vi "DialogCreateClass_HandleTemplatesDialog.vi"(8 "error in (no error)":errorcluster, 11 "AllTemplatesForThisProvider/InheritanceType(Base/Sub)":T1[](array[typedef])) -> (0 "error out":errorcluster)   [LabVIEW 2020, in "ClassWriterNative.lvclass"]
uses:
  <resource>/Framework/Providers/Open_GDS/ClassProviders/Provider_LvNativeClass/ClassWriterNative_class/ClassWriterNative.lvclass
  <resource>/Framework/Providers/Open_GDS/ClassProviders/Provider_BaseClassInterface/ClassTemplateType.ctl
  <vilib>/Utility/config.llb/Write Key (String).vi
  <vilib>/Utility/config.llb/NI_LVConfig.lvlib
  <resource>/Framework/Providers/Open_GDS/ClassProviders/Provider_BaseClassInterface/ClassWriter_class/ClassWriter.lvclass
panel:
  in  "Cancel":bool
  in  "Save":bool
  in  "Down":bool
  in  "Up":bool
  in  "ClassTemplates":i32(listbox) caption="Class Templates"
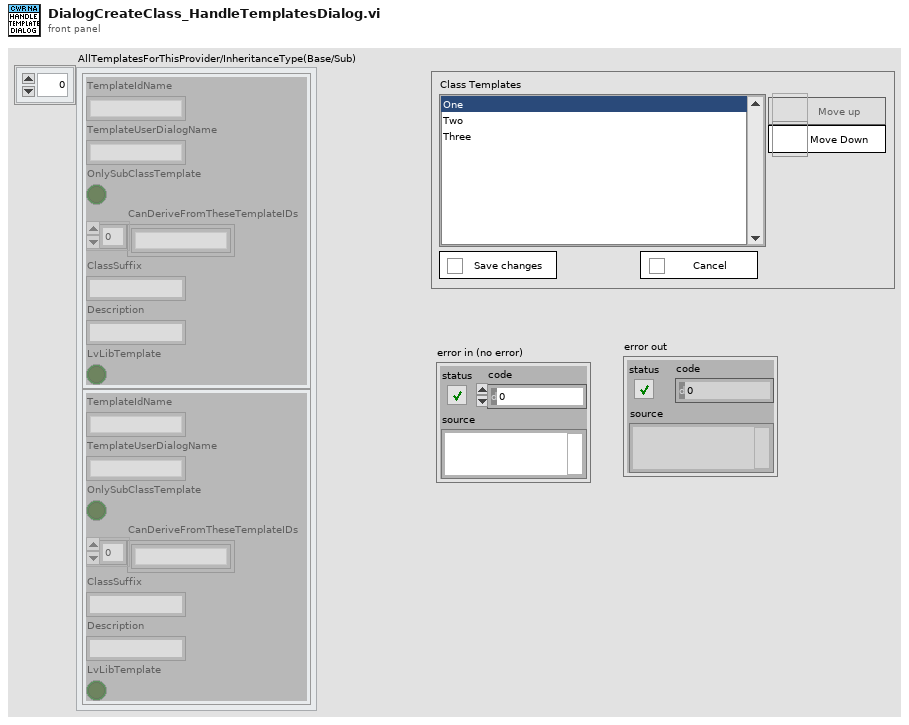
[diagram p1: front panel]
types:
  T1 = typedef "ClassWriter.lvclass/ClassTemplateType.ctl" = cluster{"TemplateIdName":string, "TemplateUserDialogName":string, "OnlySubClassTemplate":bool, "CanDeriveFromTheseTemplateIDs":string[], "ClassSuffix":string, "Description":string, "LvLibTemplate":bool}
  T2 = cluster{"FilterSettings":cluster{"Numeric":i32, "Boolean":bool}[], "Section":string}
  T3 = enum8{"Enabled", "Disabled", "Disabled and Grayed Out"}
  T4 = typedef "LVPoint32TypeDef.ctl" = cluster{"Horizontal":i32, "Vertical":i32}
  T5 = typedef "NI_LVConfig.lvlib/Config Data RefNum.ctl" = refnum<k1>
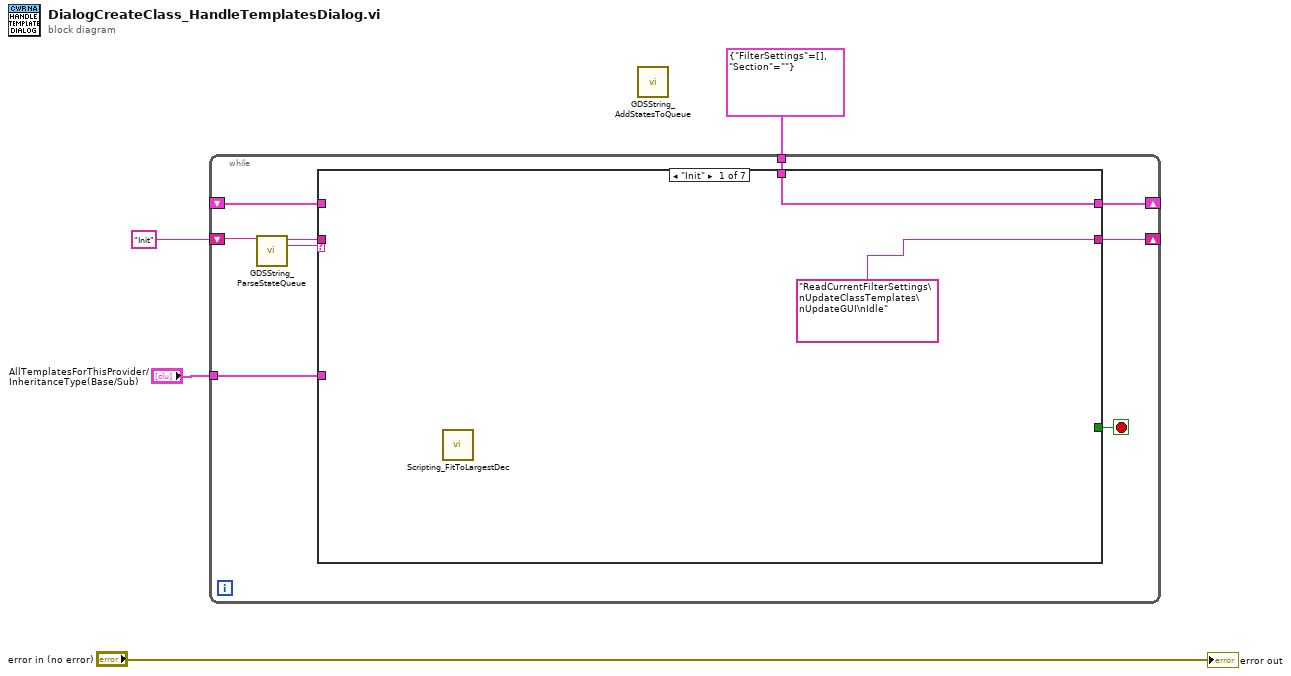
[diagram p0: block diagram]
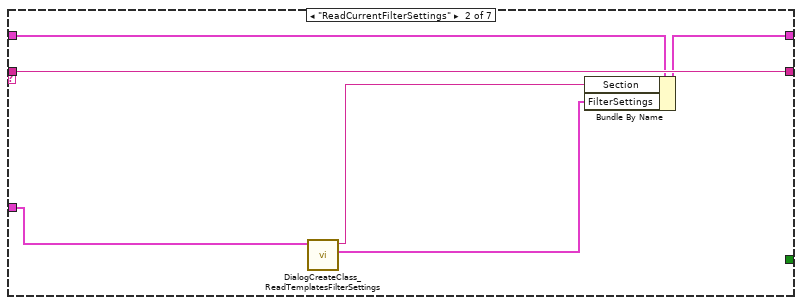
[diagram p2: hidden frame]
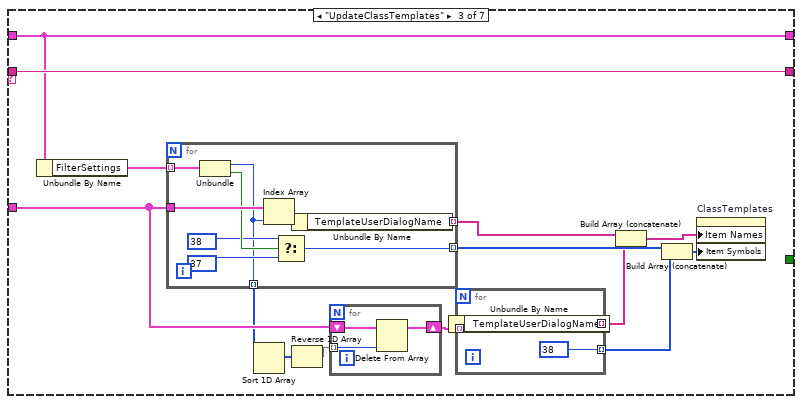
[diagram p3: hidden frame]
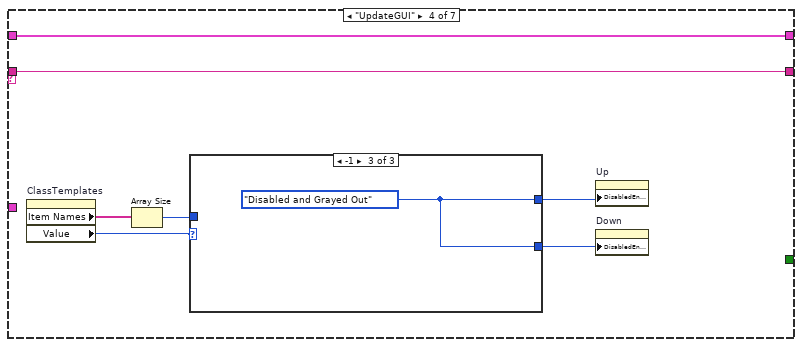
[diagram p4: hidden frame]
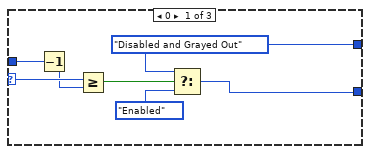
[diagram p5: hidden frame]
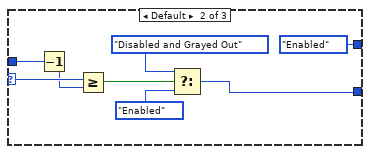
[diagram p6: hidden frame]
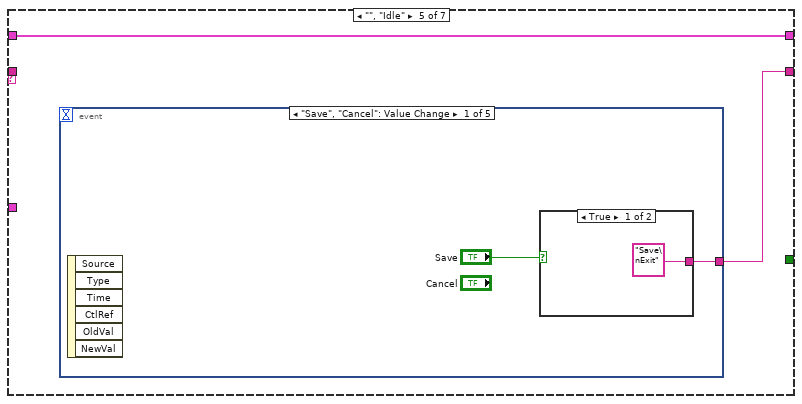
[diagram p7: hidden frame]
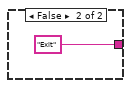
[diagram p8: hidden frame]
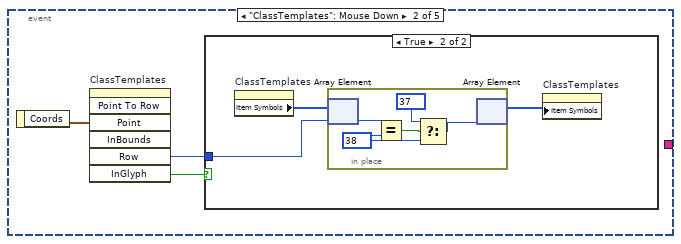
[diagram p9: hidden frame]
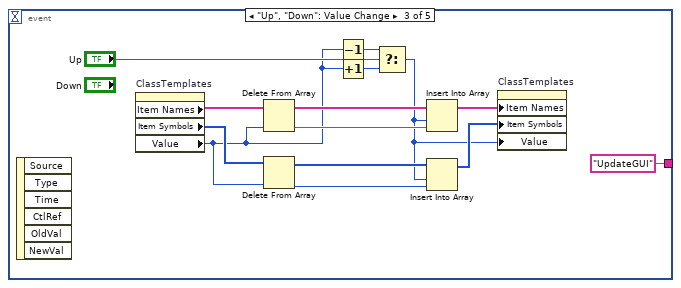
[diagram p11: hidden frame]
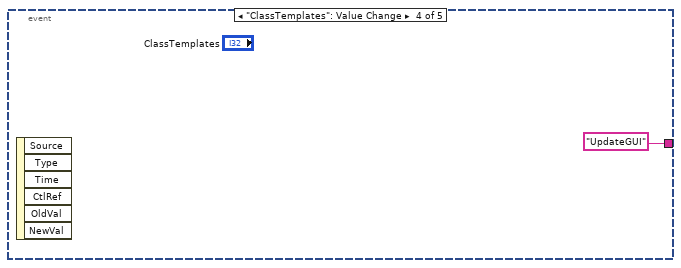
[diagram p12: hidden frame]
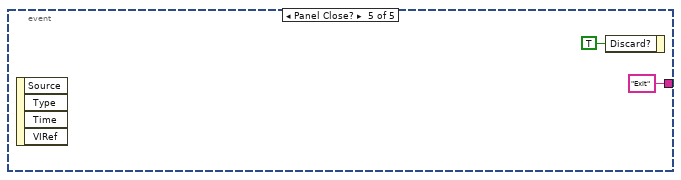
[diagram p13: hidden frame]
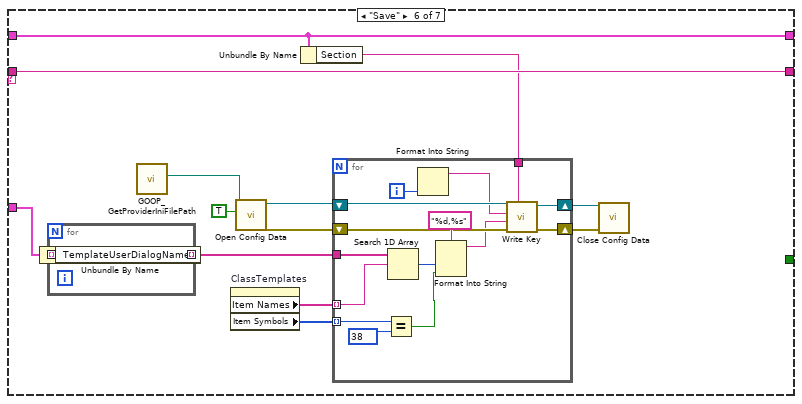
[diagram p14: hidden frame]
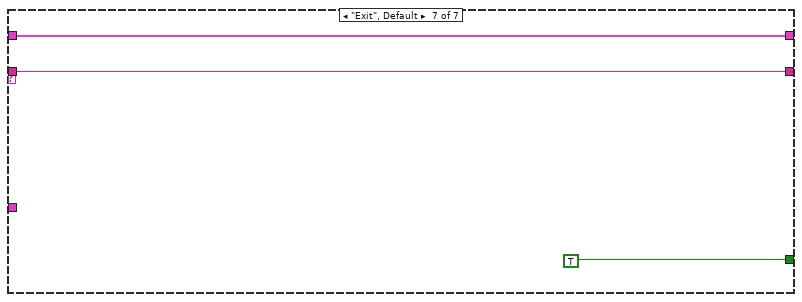
[diagram p15: hidden frame]
diagram:
  n1 = while {
    shift-right: [w11] -> _
    shift-left: "Init" -> [w12]
    tunnel: "AllTemplatesForThisProvider/InheritanceType(Base/Sub)" -> [w8]
    tunnel: T2 {"FilterSettings"=[], "Section"=""} -> [w7]
    shift-right: [w6] -> _
    shift-left: _ -> [w5]
    stop <- w13 stop-if-true
    n2 = call <resource>:"GDSString_ParseStateQueue.vi"("State Queue"=w12) -> ("Remaining States"=w9:string, "Current State"=w10:string)  [unwired: 10 in, 3 out]
    n3 = case shown="\"Init\"" w10 {
      tunnel: [_ _ _ _ _ _ TRUE] -> w13
      tunnel: ["ReadCurrentFilterSettings\nUpdateClassTemplates\nUpdateGUI\nIdle" ("Remaining States") w21 w35 w57 w75 w120 w139] -> w11
      tunnel: w9 -> [_ w21 w35 w57 _ w120 w139]
      tunnel: w8 -> [_ w20 w30 _ _ w117 _]
      tunnel: [w14 w17 w34 w56 w74 w114 w138] -> w6
      tunnel: w7 -> [w14 _ _ _ _ _ _]
      tunnel: w5 -> [_ w19 w34 w56 w74 w114 w138]
      frame "Init" {
        n4 = call <resource>:"Scripting_FitToLargestDec.vi"() -> ()  [unwired: 6 in, 2 out]
      }
      frame "ReadCurrentFilterSettings" {
        n5 = call <resource>:"DialogCreateClass_ReadTemplatesFilterSettings.vi"("AllTemplatesForThisProvider/InheritanceType(Base/Sub)"=w20) -> ("FilterSettings(OrderIndex,Active)"=w18:cluster{"Numeric":i32, "Checkbox":bool}[], "Section"=w16:string)  [unwired: 9 in]
        n6 = Bundle By Name(cluster=w19, "Section"=w16, "FilterSettings"=w18) -> (w17:T2)
      }
      frame "UpdateClassTemplates" {
        n7 = Unbundle By Name(w34) -> ("FilterSettings"=w33:cluster{"Numeric":i32, "Boolean":bool}[])
        n8 = for {
          tunnel: w33 -> [w50] mode=indexing
          tunnel: w30 -> [w49]
          tunnel: [w45] -> w32 mode=indexing
          tunnel: [w43] -> w31 mode=indexing
          tunnel: [w42] -> w29 mode=indexing
          n9 = Unbundle(w50) -> ("Numeric"=w42:i32, "Boolean"=w48:bool)
          n10 = Index Array(array=w49, index=w42) -> (element=w44:T1)
          n11 = Select(t=38, s=w48, f=37) -> (s? t:f=w45:i32)
          n12 = Unbundle By Name(w44) -> ("TemplateUserDialogName"=w43:string)
        }
        n13 = Sort 1D Array(array=w29) -> (sorted array=w28:i32[])
        n14 = Reverse 1D Array(array=w28) -> (reversed array=w27:i32[])
        n15 = for {
          shift-right: [w39] -> w26
          shift-left: w30 -> [w41]
          tunnel: w27 -> [w40] mode=indexing
          n16 = Delete From Array(array=w41, index=w40) -> (array with subset deleted=w39:T1[])  [unwired: 1 in, 1 out]
        }
        n17 = for {
          tunnel: [38] -> w22 mode=indexing
          tunnel: [w38] -> w23 mode=indexing
          tunnel: w26 -> [w36] mode=indexing
          n18 = Unbundle By Name(w36) -> ("TemplateUserDialogName"=w38:string)
        }
        n19 = Build Array (concatenate)(w31, w23) -> (w25:string[])
        n20 = Build Array (concatenate)(w32, w22) -> (w24:i32[])
        n21 = property on="ClassTemplates" class="LstBox (strict)"("Item Names"=w25, "Item Symbols"=w24) -> ()  [unwired: 2 in, 2 out]
      }
      frame "UpdateGUI" {
        n22 = property on="ClassTemplates" class="LstBox (strict)"() -> ("Item Names"=w52:string[], "Value"=w55:i32)  [unwired: 2 in, 2 out]
        n23 = Array Size(array=w52) -> (size(s)=w51:i32)
        n24 = case shown="-1" w55 {
          selector: w55 -> [w64 w72 _]
          tunnel: [w59 T3."Enabled" ("Disabled") w73] -> w54
          tunnel: [w60 w68 w73] -> w53
          tunnel: w51 -> [w63 w71 _]
          frame 0 {
            w59 = T3."Disabled and Grayed Out" ("Disabled")
            n25 = Decrement(x=w63) -> (x-1=w62:i32)
            n26 = Greater Or Equal?(x=w64, y=w62) -> (x >= y?=w61:bool)
            n27 = Select(t=w59, s=w61, f=T3."Enabled" ("Disabled")) -> (s? t:f=w60:T3)
          }
          frame Default {
            n28 = Decrement(x=w71) -> (x-1=w70:i32)
            n29 = Greater Or Equal?(x=w72, y=w70) -> (x >= y?=w69:bool)
            n30 = Select(t=T3."Disabled and Grayed Out" ("Disabled"), s=w69, f=T3."Enabled" ("Disabled")) -> (s? t:f=w68:T3)
          }
          frame -1 {
            w73 = T3."Disabled and Grayed Out" ("Disabled")
          }
        }
        n31 = property on="Up" class="Bool"("DisabledEnum"=w54) -> ()  [unwired: 2 in, 2 out]
        n32 = property on="Down" class="Bool"("DisabledEnum"=w53) -> ()  [unwired: 2 in, 2 out]
      }
      frame "", "Idle" {
        n33 = event shown="[0] \"Save\", \"Cancel\": Value Change" {
          selector: _ -> [_ _ _ _ _]
          dyn-events: _ -> [_ _ _ _ _]
          timeout: _ -> [_ _ _ _ _]
          tunnel: [w77 _ "UpdateGUI" "UpdateGUI" "Exit"] -> w75
          event "Save", "Cancel": Value Change {
            n34 = event-data() -> ()  [unwired: 1 in, 6 out]
            n35 = case shown="True" "Save" {
              tunnel: ["Save\nExit" "Exit"] -> w77
              frame True {
              }
              frame False {
              }
            }
          }
          event "ClassTemplates": Mouse Down {
            n36 = event-data() -> ("Coords"=w82:T4)  [unwired: 1 in]
            n37 = invoke on="ClassTemplates" class="LstBox (strict)" method="Point To Row"("Point"=w82) -> ("Row"=w80:i32, "InGlyph"=w81:bool)  [unwired: 6 in, 5 out]
            n38 = case shown="True" w81 {
              tunnel: w80 -> [_ w84]
              frame False {
              }
              frame True {
                n39 = property on="ClassTemplates" class="LstBox (strict)"() -> ("Item Symbols"=w85:i32[])  [unwired: 2 in, 2 out]
                n40 = in-place {
                  w88 = 38
                  n41 = in-place-array #1(w85, w84) -> (w90:i32)
                  n42 = Equal?(x=w90, y=w88) -> (x = y?=w89:bool)
                  n43 = Select(t=37, s=w89, f=w88) -> (s? t:f=w86:i32)
                  n44 = in-place-array #1(w86) -> (w83:i32[])  [unwired: 1 out]
                }
                n45 = property on="ClassTemplates" class="LstBox (strict)"("Item Symbols"=w83) -> ()  [unwired: 2 in, 2 out]
              }
            }
          }
          event "Up", "Down": Value Change {
            n46 = event-data() -> ()  [unwired: 1 in, 6 out]
            n47 = property on="ClassTemplates" class="LstBox (strict)"() -> ("Item Names"=w103:string[], "Item Symbols"=w102:i32[], "Value"=w93:i32)  [unwired: 2 in, 2 out]
            n48 = Delete From Array(array=w103, index=w93) -> (deleted portion=w99:string, array with subset deleted=w101:string[])  [unwired: 1 in]
            n49 = Delete From Array(array=w102, index=w93) -> (deleted portion=w98:i32, array with subset deleted=w100:i32[])  [unwired: 1 in]
            n50 = Decrement(x=w93) -> (x-1=w92:i32)
            n51 = Increment(x=w93) -> (x+1=w91:i32)
            n52 = Select(t=w92, s="Up", f=w91) -> (s? t:f=w94:i32)
            n53 = Insert Into Array(array=w101, index=w94, new element=w99) -> (w96:string[])
            n54 = Insert Into Array(array=w100, index=w94, new element=w98) -> (w95:i32[])
            n55 = property on="ClassTemplates" class="LstBox (strict)"("Item Names"=w96, "Item Symbols"=w95, "Value"=w94) -> ()  [unwired: 2 in, 2 out]
          }
          event "ClassTemplates": Value Change {
            n56 = event-data() -> ()  [unwired: 1 in, 6 out]
          }
          event Panel Close? {
            n57 = event-data() -> ()  [unwired: 1 in, 4 out]
            n58 = event-data("Discard?"=TRUE) -> ()  [unwired: 1 in, 1 out]
          }
        }
      }
      frame "Save" {
        n59 = for {
          tunnel: w117 -> [w122] mode=indexing
          tunnel: [w121] -> w112 mode=indexing
          n60 = Unbundle By Name(w122) -> ("TemplateUserDialogName"=w121:string)
        }
        n61 = call <resource>:"GOOP_GetProviderIniFilePath.vi"() -> ("ProviderIniPath"=w118:path)  [unwired: 10 in, 1 out]
        n62 = property on="ClassTemplates" class="LstBox (strict)"() -> ("Item Names"=w116:string[], "Item Symbols"=w111:i32[])  [unwired: 2 in, 2 out]
        n63 = call <vilib>:"Open Config Data.vi"("create file if necessary (T)"=TRUE, "configuration file path"=w118) -> ("error out"=w110:errorcluster, "refnum"=w115:T5)  [unwired: 7 in, 1 out]
        n64 = Unbundle By Name(w114) -> ("Section"=w113:string)
        n65 = for {
          tunnel: w116 -> [w134] mode=indexing
          tunnel: w113 -> [w136]
          tunnel: w112 -> [w135]
          tunnel: w111 -> [w131] mode=indexing
          shift-right: [w127] -> w108
          shift-left: w110 -> [w128]
          shift-right: [w126] -> w109
          shift-left: w115 -> [w137]
          i -> [w124]
          n66 = Equal?(x=w131, y=38) -> (x = y?=w129:bool)
          n67 = Search 1D Array(1D array=w135, element=w134) -> (index of element=w132:i32)  [unwired: 1 in]
          n68 = Format Into String(w124) -> (resulting string=w123:string)  [unwired: 3 in, 1 out]
          n69 = Format Into String(format string="%d,%s", w132, w129) -> (resulting string=w125:string)  [unwired: 2 in, 1 out]
          n70 = call-poly <vilib>:"Write Key.vi"("section"=w136, "error in (no error)"=w128, "value"=w125, "key"=w123, "refnum"=w137) -> ("error out"=w127:errorcluster, "refnum out"=w126:T5)  [unwired: 4 in, 1 out]
        }
        n71 = call <vilib>:"Close Config Data.vi"("error in (no error)"=w108, "refnum"=w109) -> ()  [unwired: 8 in, 2 out]
      }
      frame "Exit", Default {
      }
    }
  }
  n72 = call <resource>:"GDSString_AddStatesToQueue.vi"() -> ()  [unwired: 15 in, 1 out]
  "error out" <- "error in (no error)"
